vi "Convert Variant Array.vi"(10 "error in (no error)":errorcluster, 11 "Array":refnum<vi>) -> (2 "error out":errorcluster, 3 "Variant Array":variant[](array[variant]))   [LabVIEW 2020, in "Control Array.lvlib" / "ControlArray.lvclass"]
uses:
  ControlArray.lvclass
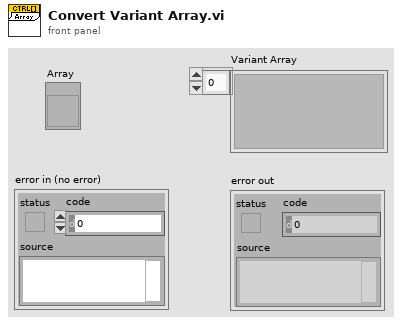
[diagram p1: front panel]
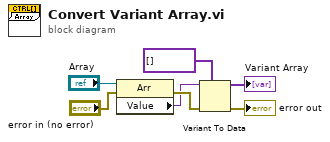
[diagram p0: block diagram]
diagram:
  n1 = property class="Arr"(reference="Array", error in="error in (no error)") -> (error out=w7:errorcluster, "Value"=w1:variant)  [unwired: 1 out]
  n2 = Variant To Data(error in=w7, type=variant[] [] ("Variant Array"), Variant=w1) -> (data=→"Variant Array":variant[], error out=→"error out":errorcluster)
